vi "ClimbQCP.vi"   [LabVIEW 2017, in "Climb.lvlib"]
uses:
  Climb.lvlib
  <userlib>/836-Library/System/QCP_V2/QCPSupportCode/QCP_GetDbl.vi
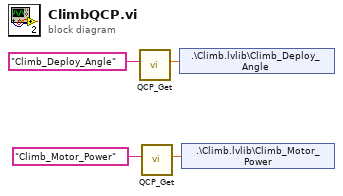
[diagram p0: block diagram]
diagram:
  n1 = call-poly <userlib>:"QCP_Get.vi"("Value Name"="Climb_Deploy_Angle") -> ("Value"=w2:dbl)  [unwired: 8 in, 2 out]
  n2 = call-poly <userlib>:"QCP_Get.vi"("Value Name"="Climb_Motor_Power") -> ("Value"=w1:dbl)  [unwired: 8 in, 2 out]
  n3 = shared-variable ".\\Climb.lvlib\\Climb_Deploy_Angle"(w2) -> ()  [unwired: 1 in, 1 out]
  n4 = shared-variable ".\\Climb.lvlib\\Climb_Motor_Power"(w1) -> ()  [unwired: 1 in, 1 out]
